vi "stiffnessGraphView.vi"(10 "UserEvents in":refnum<class "UserEvents.lvclass">) -> ()   [LabVIEW 2015, in "M1M3SSSTViews.lvlib"]
uses:
  M1M3SSSTViews.lvlib
  Typedefs/StateSelector.ctl
  Typedefs/M1M3SSSTypedefs.lvlib
  UserEvents/UserEvents.lvclass
  <vilib>/Utility/miscctls.llb/LVAnnotationListTypeDef.ctl
panel:
  out "Force vs. Distance":cluster{dbl[], dbl[]}(graph)
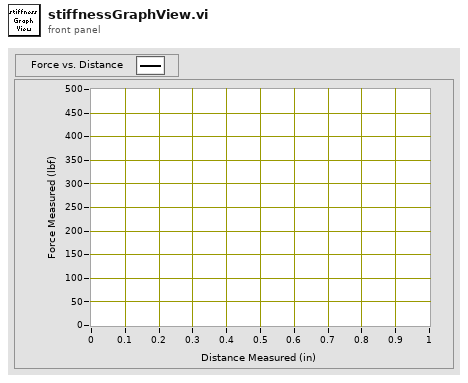
[diagram p1: front panel]
types:
  T1 = typedef "M1M3SSSTypedefs.lvlib/PubDataEvents.ctl" = cluster{"State":refnum<user-event>, "ErrorCode":refnum<user-event>, "OutputData":refnum<user-event>, "InputData":refnum<user-event>, "ControllerData":refnum<user-event>, "TestStatus":refnum<user-event>, "LogPath":refnum<user-event>, "StiffnessDataAssembly":refnum<user-event>, "PreconditioningCycle":refnum<user-event>}
  T2 = cluster{"Event Registration Refnum":refnum<event-registration>, "Event Registration Refnum":refnum<event-registration>}
  T3 = cluster{"Name":string, "Color":u32, "Style":u8, "Point Style":u8, "Name Visible":bool, "Allow Drag":bool, "Annotation Mode":u32, "Plot":i32, "Index":i32, "Position":cluster{"X":dbl, "Y":dbl}, "X Scale":u32, "Y Scale":u32, "Show Arrow":bool, "Lock Name":bool, "Plot Area":i32, "Label Offset":cluster{"X":dbl, "Y":dbl}}
  T4 = typedef "M1M3SSSTypedefs.lvlib/StateSelector.ctl" = enum16{"FaultState", "OffState", "RampingUpPressurePState", "RampingUpPressureSTState", "StandbyState", "StoppedState", "WaitingForSettledPState", "WaitingForSettledSTState"}
  T5 = typedef "LVAnnotationListTypeDef.ctl" = cluster{"Name":string, "Color":u32, "Style":u8, "Point Style":u8, "Name Visible":bool, "Allow Drag":bool, "Annotation Mode":u32, "Plot":i32, "Index":i32, "Position":cluster{"X":dbl, "Y":dbl}, "X Scale":u32, "Y Scale":u32, "Show Arrow":bool, "Lock Name":bool, "Plot Area":i32, "Label Offset":cluster{"X":dbl, "Y":dbl}}[]
  T6 = typedef "M1M3SSSTypedefs.lvlib/StiffnessData.ctl" = cluster{"Distance Measured":dbl[unit][], "Force Measured":dbl[unit][]}
  T7 = typedef "M1M3SSSTypedefs.lvlib/StiffnessesDataSummary.ctl" = cluster{"Forces":dbl[unit][], "Displacements":dbl[unit][], "Stiffnesses":dbl[unit][]}
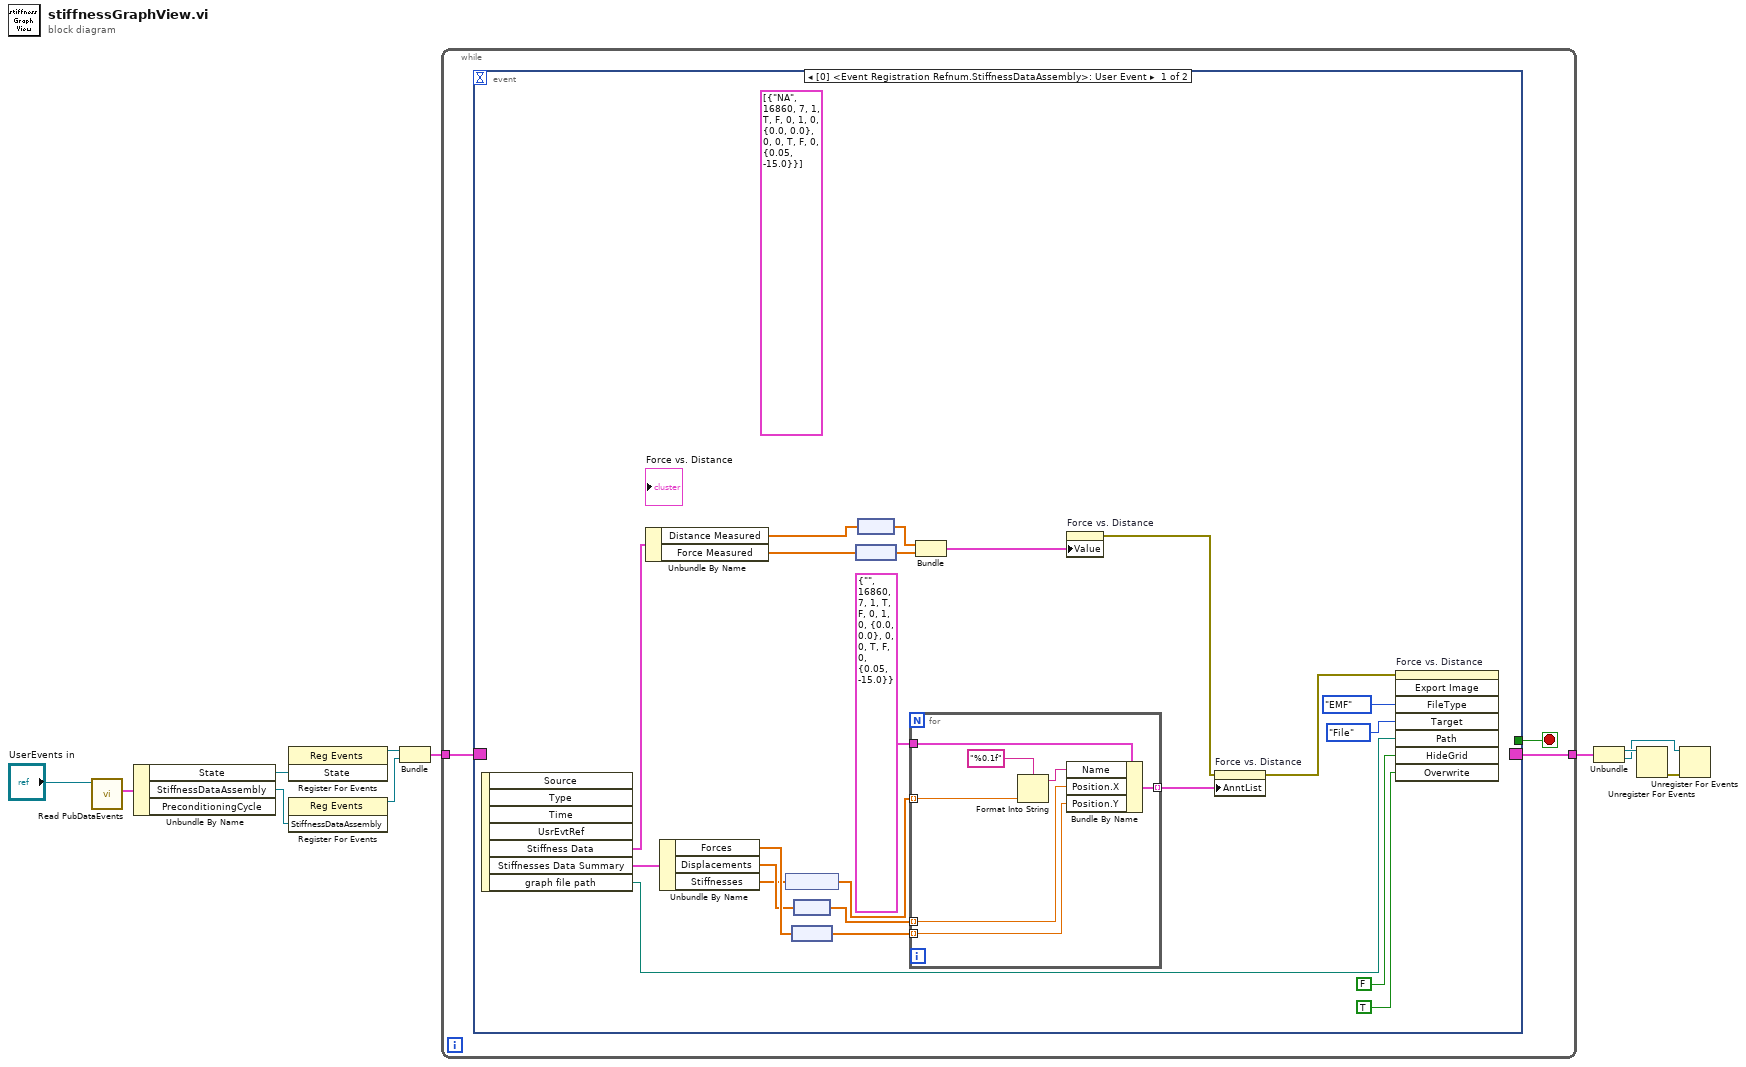
[diagram p0: block diagram]
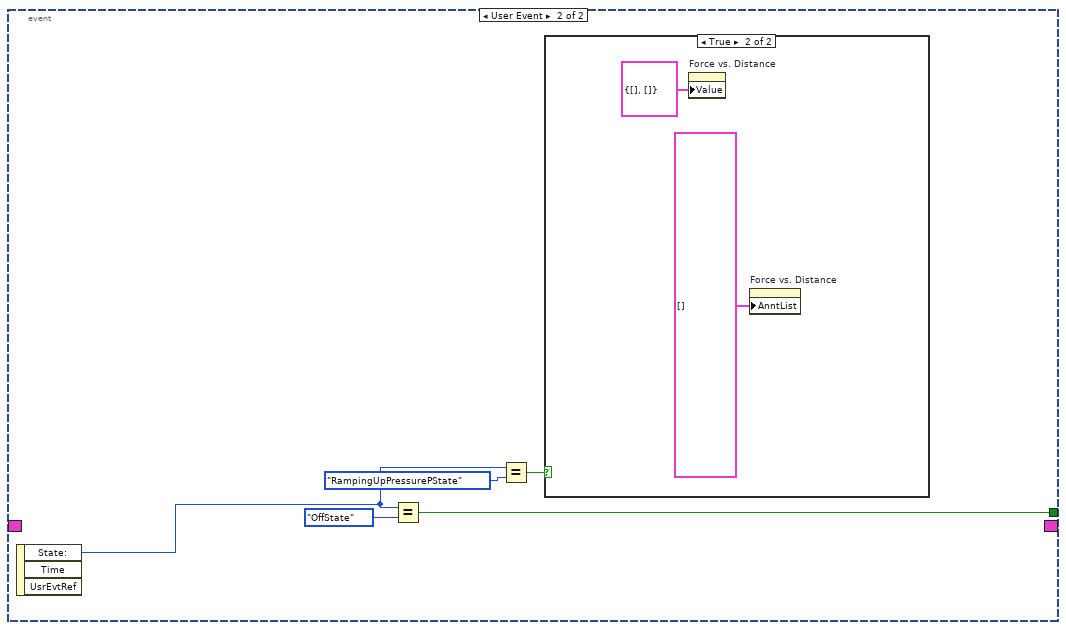
[diagram p2: hidden frame]
diagram:
  n1 = call "Read PubDataEvents.vi"("UserEvents in"="UserEvents in") -> ("PubDataEvents"=w11:T1)  [unwired: 9 in, 1 out]
  n2 = Unbundle By Name(w11) -> ("State"=w10:refnum<user-event>, "StiffnessDataAssembly"=w2:refnum<user-event>)  [unwired: 1 out]
  n3 = register-events(w10) -> (reference out=w9:refnum<event-registration>)  [unwired: 2 in, 1 out]
  n4 = register-events(w2) -> (reference out=w1:refnum<event-registration>)  [unwired: 2 in, 1 out]
  n5 = Bundle("Event Registration Refnum"=w9, "Event Registration Refnum"=w1) -> (w7:T2)  [unwired: 1 in]
  n6 = while {
    tunnel: w7 -> [w14]
    tunnel: [w12] -> w6
    stop <- w13 stop-if-true
    n7 = event shown="[0] <Event Registration Refnum.StiffnessDataAssembly>: User Event" {
      selector: w14 -> [_ _]
      dyn-events: [_ _] -> w12
      timeout: _ -> [_ _]
      tunnel: [_ w47] -> w13
      event User Event {
        (unwired) T5 [{"Name"="NA", "Color"=16860, "Style"=7, "Point Style"=1, "Name Visible"=TRUE, "Allow Drag"=FALSE, "Annotation Mode"=0, "Plot"=1, "Index"=0, "Position"={"X"=0.0, "Y"=0.0}, "X Scale"=0, "Y Scale"=0, "Show Arrow"=TRUE, "Lock Name"=FALSE, "Plot Area"=0, "Label Offset"={"X"=0.05, "Y"=-15.0}}] ("Annotation List")
        n8 = event-data() -> ("Stiffness Data"=w34:T6, "Stiffnesses Data Summary"=w31:T7, "graph file path"=w21:path)  [unwired: 1 in, 4 out]
        n9 = Unbundle By Name(w34) -> ("Distance Measured"=w33:dbl[unit][], "Force Measured"=w32:dbl[unit][])
        n10 = Unbundle By Name(w31) -> ("Forces"=w30:dbl[unit][], "Displacements"=w29:dbl[unit][], "Stiffnesses"=w28:dbl[unit][])
        n11 = node(w28) -> (w25:dbl[])
        n12 = node(w30) -> (w27:dbl[])
        n13 = node(w29) -> (w26:dbl[])
        n14 = node(w32) -> (w35:dbl[])
        n15 = node(w33) -> (w36:dbl[])
        n16 = for {
          tunnel: w26 -> [w40] mode=indexing
          tunnel: w27 -> [w39] mode=indexing
          tunnel: w25 -> [w43] mode=indexing
          tunnel: T3 {"Name"="", "Color"=16860, "Style"=7, "Point Style"=1, "Name Visible"=TRUE, "Allow Drag"=FALSE, "Annotation Mode"=0, "Plot"=1, "Index"=0, "Position"={"X"=0.0, "Y"=0.0}, "X Scale"=0, "Y Scale"=0, "Show Arrow"=TRUE, "Lock Name"=FALSE, "Plot Area"=0, "Label Offset"={"X"=0.05, "Y"=-15.0}} -> [w42]
          tunnel: [w38] -> w24 mode=indexing
          n17 = Format Into String(format string="%0.1f", w43) -> (resulting string=w41:string)  [unwired: 2 in, 1 out]
          n18 = Bundle By Name(cluster=w42, "Name"=w41, "Position.X"=w40, "Position.Y"=w39) -> (w38:T3)
        }
        n19 = Bundle(w36, w35) -> (w18:cluster{dbl[], dbl[]})  [unwired: 1 in]
        n20 = property on="Force vs. Distance" class="XYGraph (strict)"("Value"=w18) -> (error out=w17:errorcluster)  [unwired: 2 in, 1 out]
        n21 = property on="Force vs. Distance" class="XYGraph (strict)"(error in=w17, "AnntList"=w24) -> (error out=w16:errorcluster)  [unwired: 1 in, 1 out]
        n22 = invoke on="Force vs. Distance" class="XYGraph (strict)" method="Export Image"(error in=w16, "FileType"=enum32{"BMP", "EPS", "EMF", "PICT"}."EMF" ("File Type"), "Target"=enum32{"File", "Clipboard"}."File", "Path"=w21, "HideGrid"=FALSE, "Overwrite"=TRUE ("Always Overwrite")) -> ()  [unwired: 2 in, 8 out]
      }
      event User Event {
        n23 = event-data() -> ("State:"=w45:T4)  [unwired: 1 in, 2 out]
        n24 = Equal?(x=w45, y=StateSelector."OffState" ("State:")) -> (x = y?=w47:bool)
        n25 = Equal?(x=w45, y=StateSelector."RampingUpPressurePState" ("State:")) -> (x = y?=w44:bool)
        n26 = case shown="True" w44 {
          frame False {
          }
          frame True {
            n27 = property on="Force vs. Distance" class="XYGraph (strict)"("Value"=cluster{dbl[], dbl[]} {[], []} ("Force vs. Distance")) -> ()  [unwired: 2 in, 2 out]
            n28 = property on="Force vs. Distance" class="XYGraph (strict)"("AnntList"=T5 [] ("Annotation List")) -> ()  [unwired: 2 in, 2 out]
          }
        }
      }
    }
  }
  n29 = Unbundle(w6) -> ("Event Registration Refnum"=w5:refnum<event-registration>, "Event Registration Refnum"=w4:refnum<event-registration>)
  n30 = Unregister For Events(event registration refnum=w5) -> (error out=w3:errorcluster)  [unwired: 1 in]
  n31 = Unregister For Events(event registration refnum=w4, error in=w3) -> ()  [unwired: 1 out]
